vi "Listener.vi"(8 "error in (no error)":errorcluster, 11 "Gen 2 in":refnum<class "Gen 2.lvclass">) -> (0 "error out":errorcluster, 2 "Buffer Dump":string, 3 "Gen 2 out":refnum<class "Gen 2.lvclass">)   [LabVIEW 2018, in "Gen 2.lvlib" / "Gen 2.lvclass"]
uses:
  Gen 2.lvclass
  PPLs/Laser/Parent/Laser.lvlibp/Laser.lvclass
  C:/Projects/LabVIEW/PPLs/Laser/Parent/Laser.lvlibp/Laser.lvclass
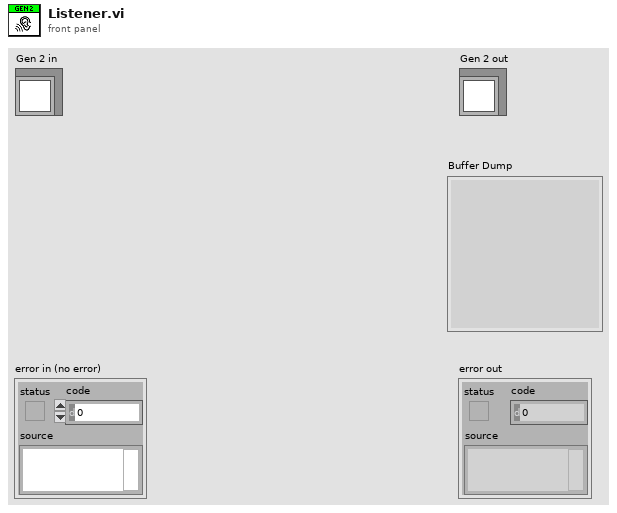
[diagram p1: front panel]
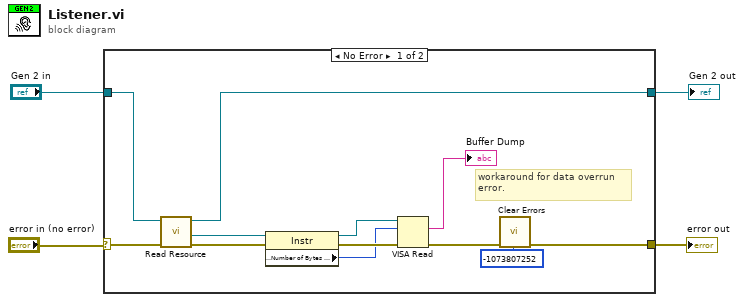
[diagram p0: block diagram]
diagram:
  n1 = case shown="No Error" "error in (no error)" {
    selector: "error in (no error)" -> [w15 w17]
    tunnel: "Gen 2 in" -> [w16 w18]
    tunnel: [w14 w18] -> w1
    tunnel: [w8 w17] -> w2
    frame No Error {
      # "workaround for data overrun\nerror."
      n2 = call "Read Resource.vi"("error in (no error)"=w15, "Laser in"=w16) -> ("error out"=w7:errorcluster, "Resource"=w6:refnum<visa-resource-name>, "Laser out"=w14:refnum<class "Gen 2.lvclass">)  [unwired: 7 in]
      n3 = property class="Instr"(reference=w6, error in=w7) -> (reference out=w12:refnum<visa-resource-name>, error out=w13:errorcluster, "Serial Settings:Number of Bytes at Serial Port"=w11:u32)
      n4 = VISA Read(VISA resource name=w12, byte count=w11, error in (no error)=w13) -> (read buffer=→"Buffer Dump":string, error out=w10:errorcluster)  [unwired: 2 out]
      n5 = call <vilib>:"Clear Errors.vi"("error in (no error)"=w10, "specific error code to clear (0: all)"=-1073807252) -> ("error out"=w8:errorcluster)  [unwired: 4 in, 1 out]
    }
    frame Error {
    }
  }
  "error out" <- w2
  "Gen 2 out" <- w1
